vi "Save.vi"(8 "error in (no error)":errorcluster, 9 "new command":string, 10 "Msg in":T1, 11 "FakePressureController in":refnum<class "MagAnalysis_Online.lvclass">) -> (0 "error out":errorcluster, 1 "Path":path, 2 "Msg out":T1, 3 "FakePressureController out":refnum<class "MagAnalysis_Online.lvclass">, 4 "new command":string)   [LabVIEW 2013, in "MagAnalysis_Online.lvclass"]
uses:
  MagAnalysis_Online.lvclass
  DriverMsg.ctl
  MagAnalysis_Online.lvclass/MagAnalysis_Online.ctl
  DaqPad_NI6009.lvclass
panel:
  out "error out 2":errorcluster
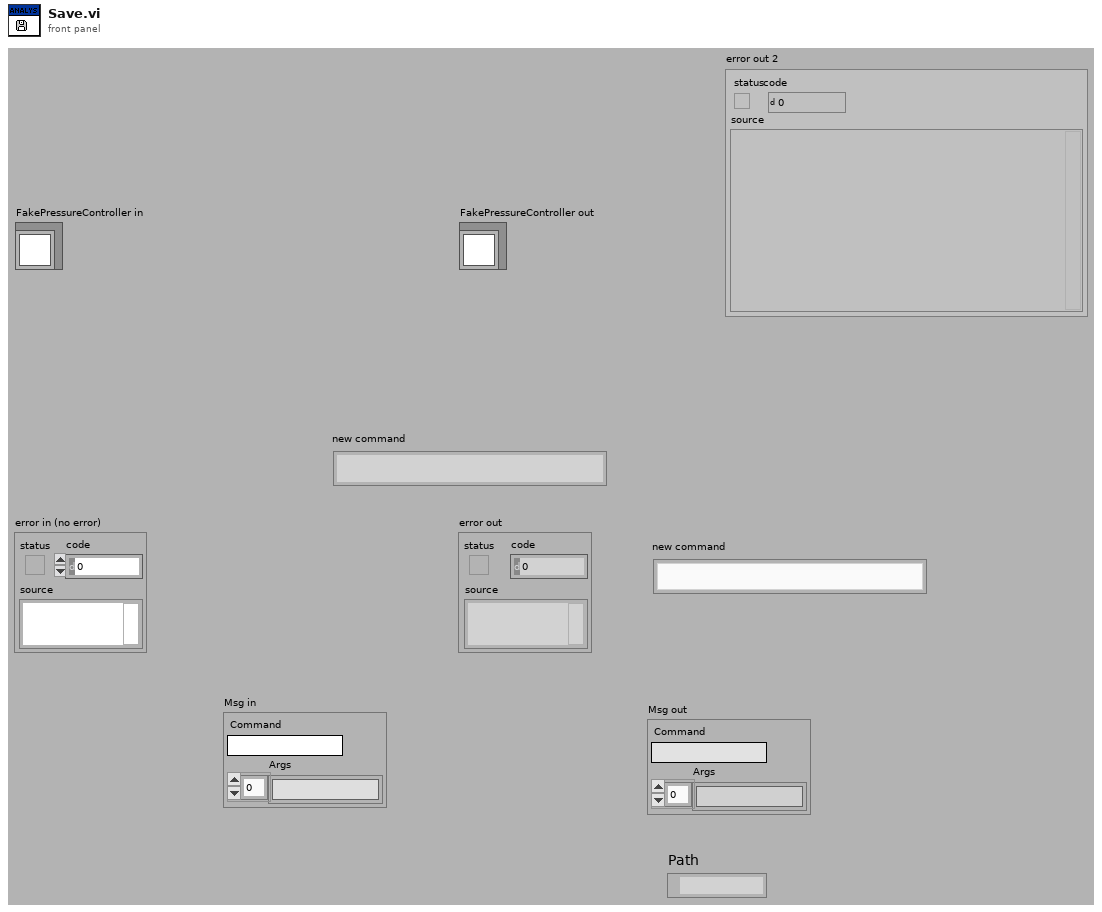
[diagram p1: front panel]
types:
  T1 = typedef "DriverMsg.ctl" = cluster{"Command":string, "Args":string[]}
  T2 = typedef "IMAQ Image.ctl" = refnum<image>
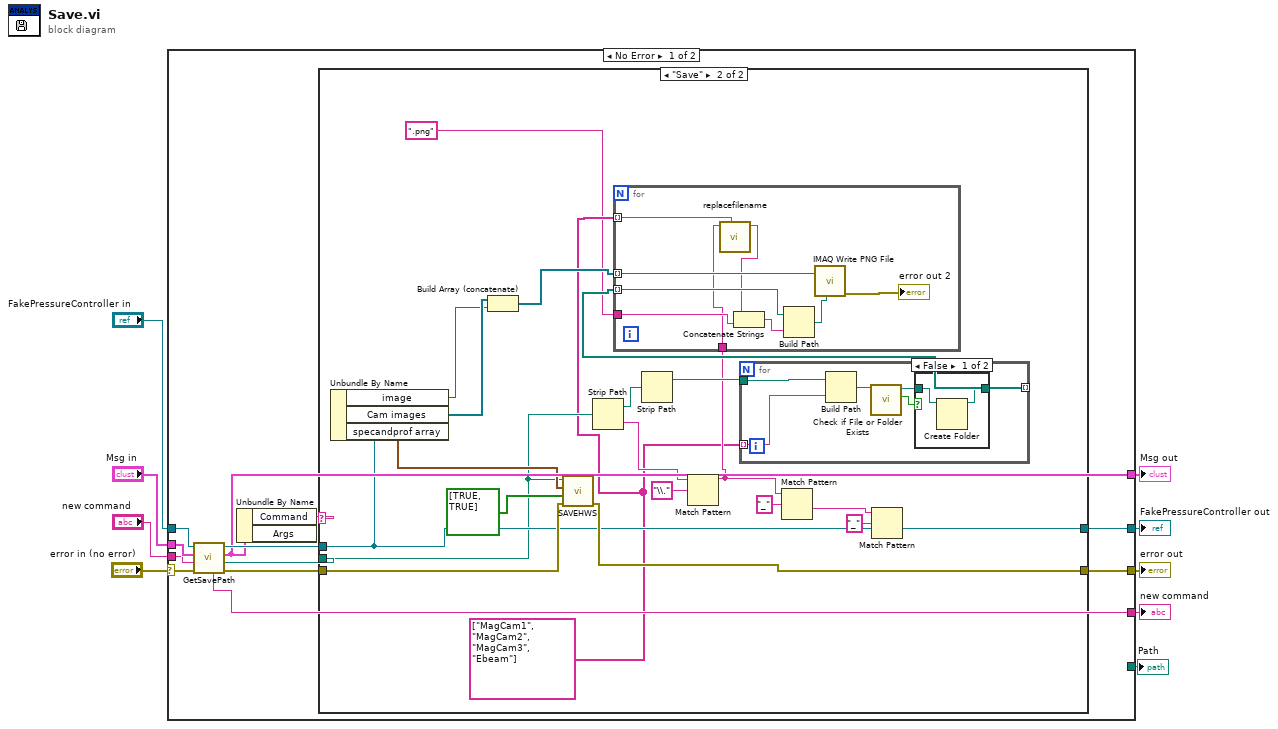
[diagram p0: block diagram]
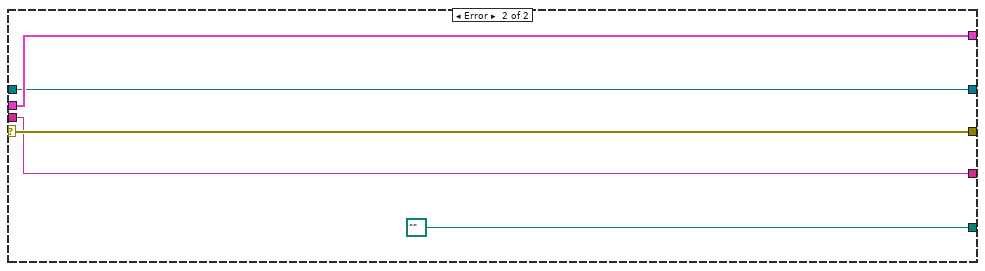
[diagram p4: hidden frame]
diagram:
  n1 = case shown="No Error" "error in (no error)" {
    selector: "error in (no error)" -> [w15 w66]
    tunnel: [w19 w66] -> w5
    tunnel: [_ path "" ("Path")] -> w1
    tunnel: [w13 w65] -> w6
    tunnel: [w20 w64] -> w8
    tunnel: "Msg in" -> [w17 w65]
    tunnel: "FakePressureController in" -> [w18 w64]
    tunnel: "new command" -> [w16 w62]
    tunnel: [w10 w62] -> w2
    frame No Error {
      n2 = call-dynamic "GetSavePath.vi"("error in (no error)"=w15, "new command"=w16, "Msg in"=w17, "BaseDriver in"=w18) -> ("error out"=w11:errorcluster, "Path"=w12:path, "Msg out"=w13:T1, "BaseDriver out"=w14:refnum<class "MagAnalysis_Online.lvclass">, "new command"=w10:string)  [unwired: 3 in]
      n3 = Unbundle By Name(w13) -> ("Command"=w21:string)  [unwired: 1 out]
      n4 = case shown="\"Save\"" w21 {
        tunnel: w14 -> [w23 w40]
        tunnel: [w23 w40] -> w20
        tunnel: w12 -> [_ w38]
        tunnel: w11 -> [w22 w42]
        tunnel: [w22 w41] -> w19
        frame Default {
        }
        frame "Save" {
          w25 = string[] ["MagCam1", "MagCam2", "MagCam3", "Ebeam"]
          n5 = Unbundle By Name(w40) -> ("image"=w32:T2, "Cam images"=w33:T2[], "specandprof array"=w39:waveform(dbl)[])
          n6 = Build Array (concatenate)(w33, w32) -> (w31:T2[])
          n7 = call "SAVEHWS.vi"("error in (no error)"=w42, "Enable (Array)"=bool[] [TRUE, TRUE], "data"=w39, "Destination HWS File"=w38) -> ("error out"=w41:errorcluster)  [unwired: 7 in]
          n8 = Strip Path(path=w38) -> (stripped path=w34:path, name=w30:string)
          n9 = Strip Path(path=w34) -> (stripped path=w36:path)  [unwired: 1 out]
          n10 = Match Pattern(string=w30, regular expression="\\.") -> (before substring=w29:string)  [unwired: 1 in, 3 out]
          n11 = for {
            tunnel: w36 -> [w49]
            tunnel: w25 -> [w48] mode=indexing
            tunnel: [w44] -> w35 mode=indexing
            n12 = Build Path(base path=w49, name or relative path=w48) -> (appended path=w47:path)
            n13 = call "Check if File or Folder Exists.vi"("path"=w47) -> ("file or folder exists?"=w45:bool, "dup path"=w46:path)  [unwired: 8 in, 1 out]
            n14 = case shown="False" w45 {
              tunnel: w46 -> [w51 w52]
              tunnel: [w50 w52] -> w44
              frame False {
                n15 = Create Folder(path (use dialog)=w51) -> (created path=w50:path)  [unwired: 2 in, 2 out]
              }
              frame True {
              }
            }
          }
          n16 = for {
            tunnel: w35 -> [w58] mode=indexing
            tunnel: ".png" ("string") -> [w57]
            tunnel: w31 -> [w56] mode=indexing
            tunnel: w29 -> [w55]
            tunnel: w25 -> [w53] mode=indexing
            n17 = call "replacefilename.vi"("new filenamePART"=w53, "filename"=w55) -> ("filename out"=w54:string)  [unwired: 9 in]
            n18 = Concatenate Strings(w54, w57) -> (w59:string)
            n19 = Build Path(base path=w58, name or relative path=w59) -> (appended path=w60:path)
            n20 = call "IMAQ Write PNG File"("File Path"=w60, "Image"=w56) -> ("error out"=→"error out 2":errorcluster)  [unwired: 4 in, 2 out]
          }
          n21 = Match Pattern(string=w29, regular expression="_") -> (after substring=w26:string)  [unwired: 1 in, 3 out]
          n22 = Match Pattern(string=w26, regular expression="_") -> ()  [unwired: 1 in, 4 out]
        }
      }
    }
    frame Error {
    }
  }
  "error out" <- w5
  "FakePressureController out" <- w8
  "Path" <- w1
  "Msg out" <- w6
  "new command" <- w2
